vi "Labspec Save.vi"(6 "ID":i32, 7 "Format":u16(ring) items=["default", "ngs - Labspec", "ngc - Labspec", "ngv - Labspec", "tsf - Labspec", "ms0 - Dilor", "ss0 - Dilor", "spc - Grams", "tif - Image", "bmp - Image", "jpg - Image", "txt - Text"], 8 "error in":errorcluster, 9 "Path":path, 10 "Filename":string, 11 "Automation Refnum In":refnum<k7>) -> (0 "error out":errorcluster, 1 "File Path":path, 3 "Automation Refnum Out":refnum<k7>)   [LabVIEW 2014]
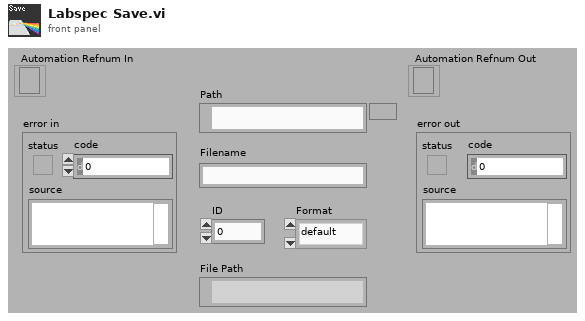
[diagram p1: front panel]
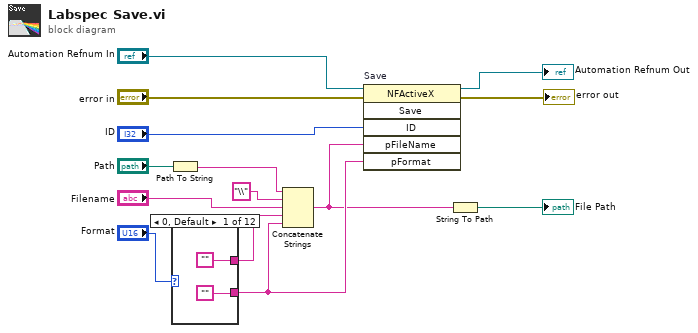
[diagram p0: block diagram]
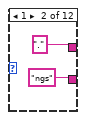
[diagram p2: hidden frame]
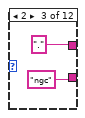
[diagram p3: hidden frame]
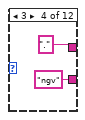
[diagram p4: hidden frame]
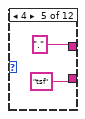
[diagram p5: hidden frame]
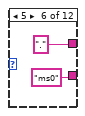
[diagram p6: hidden frame]
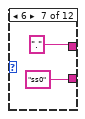
[diagram p7: hidden frame]
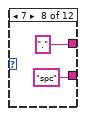
[diagram p8: hidden frame]
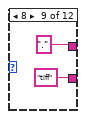
[diagram p9: hidden frame]
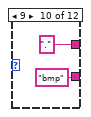
[diagram p10: hidden frame]
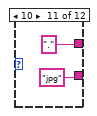
[diagram p11: hidden frame]
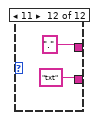
[diagram p12: hidden frame]
diagram:
  n1 = Path To String(path="Path") -> (string=w3:string)
  n2 = case shown="0, Default" "Format" {
    tunnel: ["" "ngs" "ngc" "ngv" "tsf" "ms0" "ss0" "spc" "tiff" "bmp" "jpg" "txt"] -> w7
    tunnel: ["" "." "." "." "." "." "." "." "." "." "." "."] -> w8
    frame 0, Default {
    }
    frame 1 {
    }
    frame 2 {
    }
    frame 3 {
    }
    frame 4 {
    }
    frame 5 {
    }
    frame 6 {
    }
    frame 7 {
    }
    frame 8 {
    }
    frame 9 {
    }
    frame 10 {
    }
    frame 11 {
    }
  }
  n3 = Concatenate Strings(w3, "\\" ("string"), "Filename", w8, w7) -> (w2:string)
  n4 = invoke on="Save" class="NFActiveX" method="Save"(reference="Automation Refnum In", error in="error in", "ID"="ID", "pFileName"=w2, "pFormat"=w7) -> (reference out=→"Automation Refnum Out":refnum<k7>, error out=→"error out":errorcluster)  [unwired: 1 in, 4 out]
  n5 = String To Path(string=w2) -> (path=→"File Path":path)
